vi "Untitled 1.vi"() -> ()   [LabVIEW 2025, in "phlair-busch-can-bus.lvlib"]
uses:
  phlair-busch-can-bus.lvlib
  <vilib>/xnet/xnet.llb/XNET Read (Signal Single-point).vi
panel:
  out "error out":errorcluster
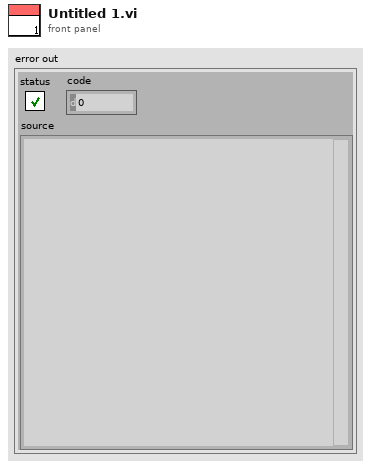
[diagram p1: front panel]
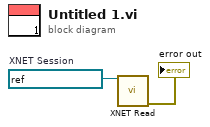
[diagram p0: block diagram]
diagram:
  w2 = refnum<k21> "Sess_Actuals"  # XNET Session
  n1 = call-poly <vilib>:"XNET Read.vi"("session in"=w2) -> ("error out"=→"error out":errorcluster)  [unwired: 12 in, 2 out]
